vi "swish and swipe.vi"() -> ()   [LabVIEW 2020]
uses:
  <vilib>/Instr/_visa.llb/VISA Configure Serial Port (Instr).vi
panel:
  out "TWIST":bool
  out "SWISH":bool
  out "SWIPIE":bool
  out "SD Z":dbl format="%0.2f"
  out "SD Y":dbl format="%0.2f"
  out "SD X":dbl format="%0.2f"
  out "x > y?":bool
  out "Angle Z":dbl
  out "Angle Y":dbl
  out "Angle X":dbl
  out "Waveform Chart 5":cluster{"wx":dbl, "wy":dbl, "wz":dbl}(graph)
  in  "Stop Button":bool
  out "Console":string
  in  "Data to write":string
  in  "VISA resource name":refnum<visa-resource-name>
  # "01 Talking Serial\nThis code is a very simple terminal emulator\n\nInstructions:\n1. Select the desired serial port\n2. Hit Run and try it out (note that it will send your text and a '\\n')"
  # "Hit return when done typing"
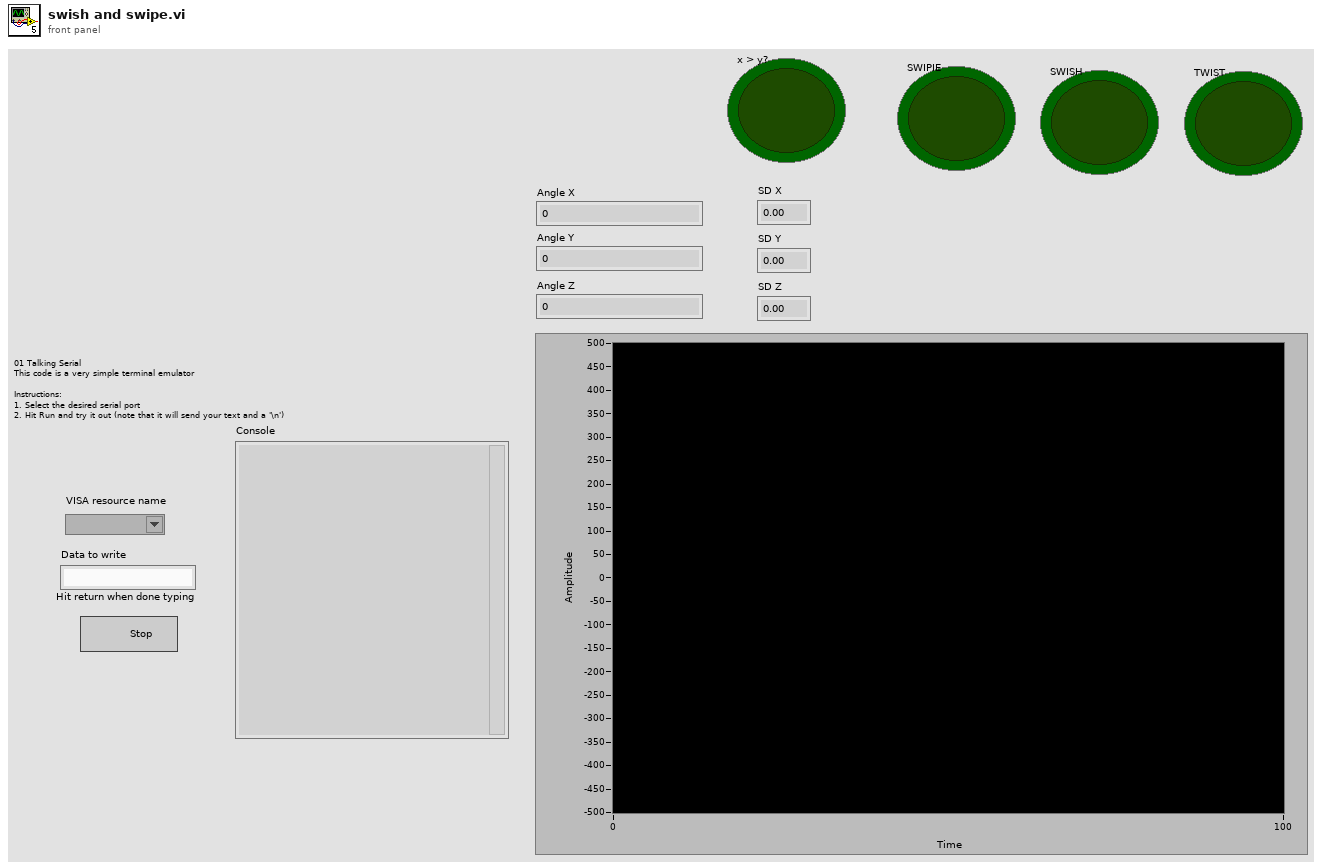
[diagram p1: front panel]
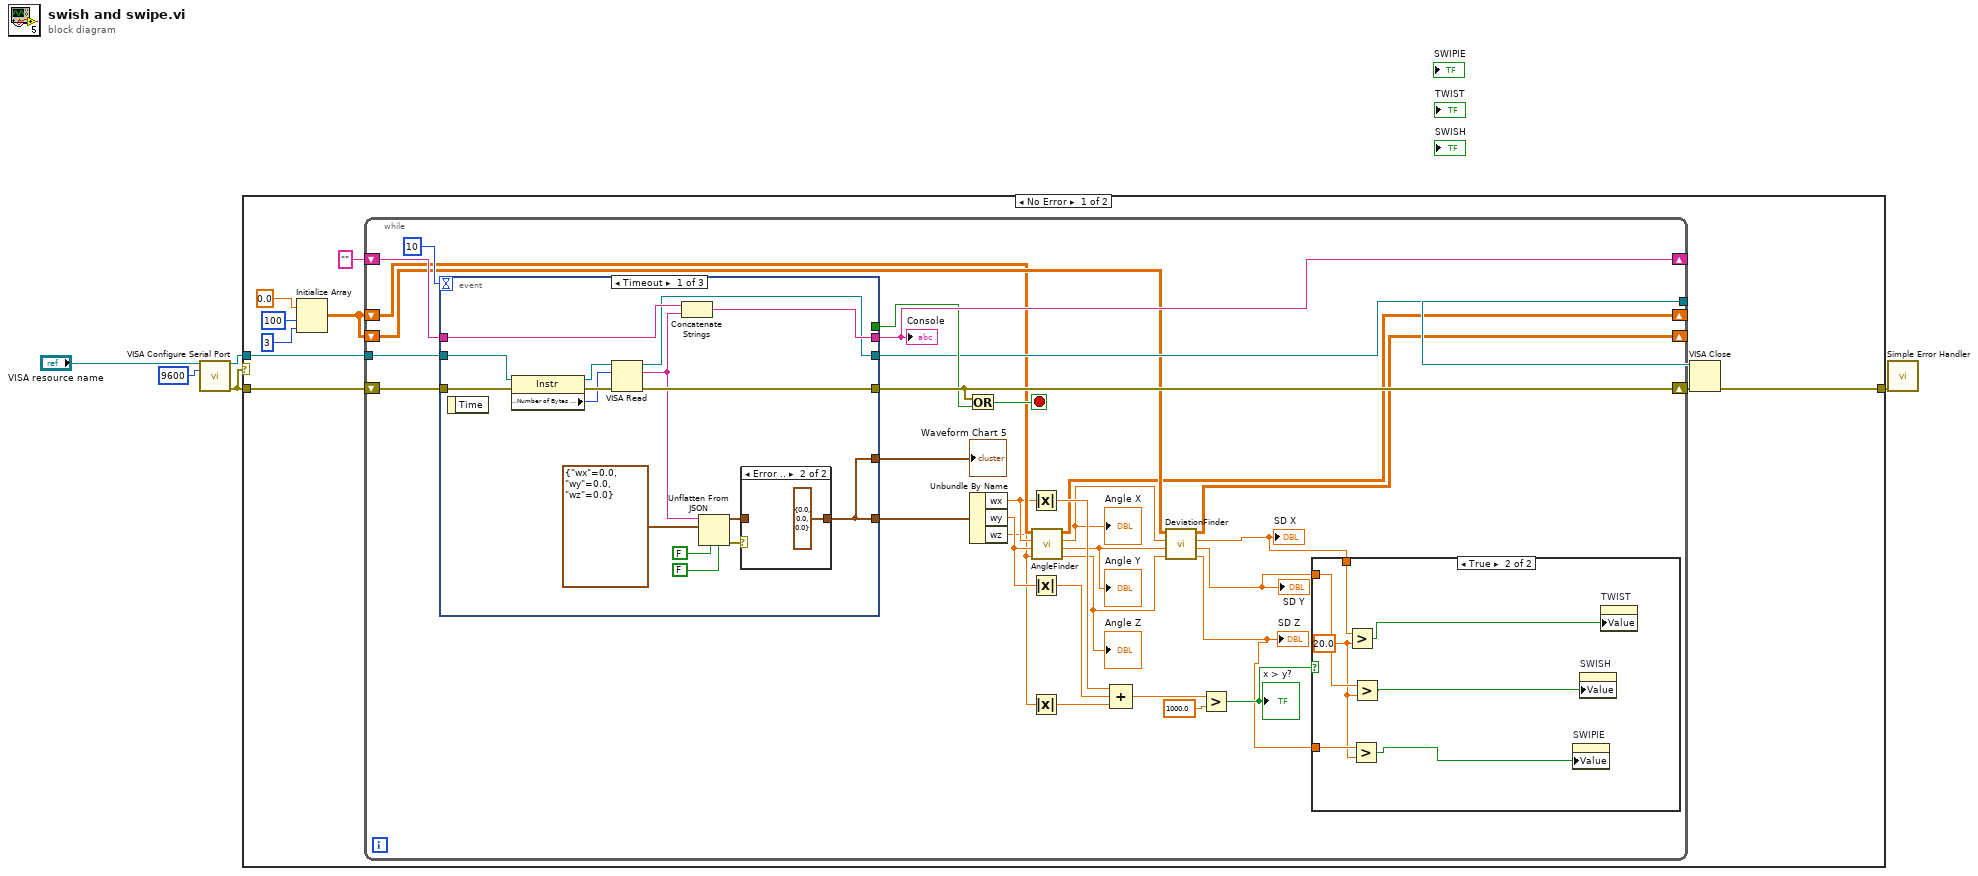
[diagram p0: block diagram]
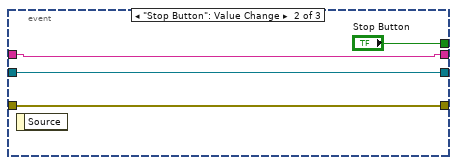
[diagram p4: hidden frame]
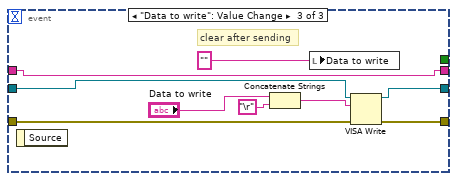
[diagram p5: hidden frame]
diagram:
  n1 = call-poly "VISA Configure Serial Port"("VISA resource name"="VISA resource name", "baud rate (9600)"=u32 9600) -> ("VISA resource name out"=w3:refnum<visa-resource-name>, "error out"=w2:errorcluster)  [unwired: 12 in]
  n2 = case shown="No Error" w2 {
    tunnel: w3 -> [w15 _]
    tunnel: w2 -> [w14 w84]
    tunnel: [w10 w84] -> w1
    frame No Error {
      n3 = Initialize Array(0.0 ("element"), 100 ("dimension size"), 3 ("dimension size")) -> (w6:dbl[][])
      n4 = while {
        tunnel: w15 -> [w45]
        shift-right: [w40] -> w11
        shift-left: w14 -> [w44]
        shift-right: [w41] -> _
        shift-left: "" -> [w42]
        tunnel: [w37] -> w12
        shift-right: [w28] -> _
        shift-left: w6 -> [w30]
        shift-right: [w29] -> _
        shift-left: w6 -> [w26]
        stop <- w38 stop-if-true
        n5 = event shown="[0] Timeout" {
          selector: _ -> [_ _ _]
          dyn-events: _ -> [_ _ _]
          timeout: 10 -> [_ _ _]
          tunnel: w45 -> [w68 w71 w83]
          tunnel: w44 -> [w67 w73 w82]
          tunnel: [w63 w73 w81] -> w40
          tunnel: w42 -> [w62 w72 w80]
          tunnel: [w61 w72 w80] -> w41
          tunnel: [_ "Stop Button" _] -> w39
          tunnel: [w60 w71 w78] -> w37
          tunnel: [w53 _ _] -> w36
          tunnel: [w53 _ _] -> w27
          event Timeout {
            n6 = event-data() -> ()  [unwired: 1 in, 1 out]
            n7 = property class="Instr"(reference=w68, error in=w67) -> (reference out=w64:refnum<visa-resource-name>, error out=w66:errorcluster, "Serial Settings:Number of Bytes at Serial Port"=w65:u32)
            n8 = VISA Read(VISA resource name=w64, byte count=w65, error in (no error)=w66) -> (VISA resource name out=w60:refnum<visa-resource-name>, read buffer=w59:string, error out=w63:errorcluster)  [unwired: 1 out]
            n9 = Concatenate Strings(w62, w59) -> (w61:string)
            n10 = Unflatten From JSON(JSON string=w59, type and defaults=cluster{"wx":dbl, "wy":dbl, "wz":dbl} {"wx"=0.0, "wy"=0.0, "wz"=0.0}, default null elements? (F)=FALSE, strict validation? (F)=FALSE) -> (value=w54:cluster{"wx":dbl, "wy":dbl, "wz":dbl}, error out=w55:errorcluster)  [unwired: 3 in]
            n11 = case shown="Error .." w55 {
              tunnel: [w69 cluster{"wx":dbl, "wy":dbl, "wz":dbl} {"wx"=0.0, "wy"=0.0, "wz"=0.0}] -> w53
              tunnel: w54 -> [w69 _]
              frame No Error {
              }
              frame Error {
              }
            }
          }
          event "Stop Button": Value Change {
            n12 = event-data() -> ()  [unwired: 1 in, 1 out]
          }
          event "Data to write": Value Change {
            # "clear after sending"
            n13 = event-data() -> ()  [unwired: 1 in, 1 out]
            n14 = Concatenate Strings("Data to write", "\r") -> (w76:string)
            n15 = local write "Data to write"("" ("Data to write")) -> ()
            n16 = VISA Write(VISA resource name=w83, write buffer=w76, error in (no error)=w82) -> (VISA resource name out=w78:refnum<visa-resource-name>, error out=w81:errorcluster)  [unwired: 1 out]
          }
        }
        "Console" <- w41
        "Waveform Chart 5" <- w36
        n17 = Or(x=w40, y=w39) -> (x .or. y?=w38:bool)
        n18 = Unbundle By Name(w27) -> ("wx"=w22:dbl, "wy"=w21:dbl, "wz"=w20:dbl)
        n19 = Absolute Value(x=w22) -> (abs(x)=w35:dbl)
        n20 = Absolute Value(x=w21) -> (abs(x)=w34:dbl)
        n21 = Absolute Value(x=w20) -> (abs(x)=w33:dbl)
        n22 = call "AngleFinder.vi"("wz"=w20, "wy"=w21, "wx"=w22, "Array in"=w26) -> ("Z"=w23:dbl, "Y"=w24:dbl, "X"=w25:dbl, "Array out"=w29:dbl[][])  [unwired: 4 in]
        "Angle X" <- w25
        "Angle Y" <- w24
        "Angle Z" <- w23
        n23 = Compound Arithmetic op=ADD(w35, w34, w33) -> (w31:dbl)
        n24 = call "DeviationFinder.vi"("Z"=w23, "Y"=w24, "X"=w25, "Array in"=w30) -> ("SD Z"=w16:dbl, "SD Y"=w17:dbl, "SD X"=w18:dbl, "Array out"=w28:dbl[][])  [unwired: 4 in]
        "SD X" <- w18
        "SD Y" <- w17
        "SD Z" <- w16
        n25 = Greater?(x=w31, y=1000.0) -> (0:w19:bool)
        "x > y?" <- w19
        n26 = case shown="True" w19 {
          tunnel: w18 -> [_ w52]
          tunnel: w17 -> [_ w51]
          tunnel: w16 -> [_ w50]
          frame False {
          }
          frame True {
            w49 = 20.0 ("y")
            n27 = Greater?(x=w52, y=w49) -> (0:w46:bool)
            n28 = Greater?(x=w50, y=w49) -> (0:w48:bool)
            n29 = Greater?(x=w51, y=w49) -> (0:w47:bool)
            n30 = property on="SWIPIE" class="Bool (strict)"("Value"=w48) -> ()  [unwired: 2 in, 2 out]
            n31 = property on="SWISH" class="Bool (strict)"("Value"=w47) -> ()  [unwired: 2 in, 2 out]
            n32 = property on="TWIST" class="Bool (strict)"("Value"=w46) -> ()  [unwired: 2 in, 2 out]
          }
        }
      }
      n33 = VISA Close(VISA resource name=w12, error in (no error)=w11) -> (error out=w10:errorcluster)
    }
    frame Error {
    }
  }
  n34 = call <vilib>:"Simple Error Handler.vi"("error in (no error)"=w1) -> ()  [unwired: 4 in, 5 out]
